vi "pmu_Build Time Quality (Std 2011).vi"(0 "reported GPS information":T1, 1 "max time error [s]":dbl=1e-07 format="%#_15f", 9 "system info in":refnum<class "PMU System Info.lvclass">, 11 "error in (no error)":errorcluster) -> (4 "reporting timing information":T2 {"PMU time quality" format="%.0b"; "time quality flag" format="%.0b"}, 10 "system info out":refnum<class "PMU System Info.lvclass">, 15 "error out":errorcluster)   [LabVIEW 2015, in "NI_EP_PMU.lvlib"]
doc: "Outputs time quality flag bits, according to IEEE Std C37.118."
uses:
  <vilib>/addons/Electrical Power/PMU/NI_EP_PMU.lvlib
  <vilib>/addons/Electrical Power/PMU/Common/Controls/pmu_Reporting Time Information (Std 2011).ctl
  <vilib>/addons/Electrical Power/PMU/Common/Classes/PMU System Info/PMU System Info.lvclass
  <vilib>/addons/Electrical Power/PMU/Common/Controls/pmu_GPS Info.ctl
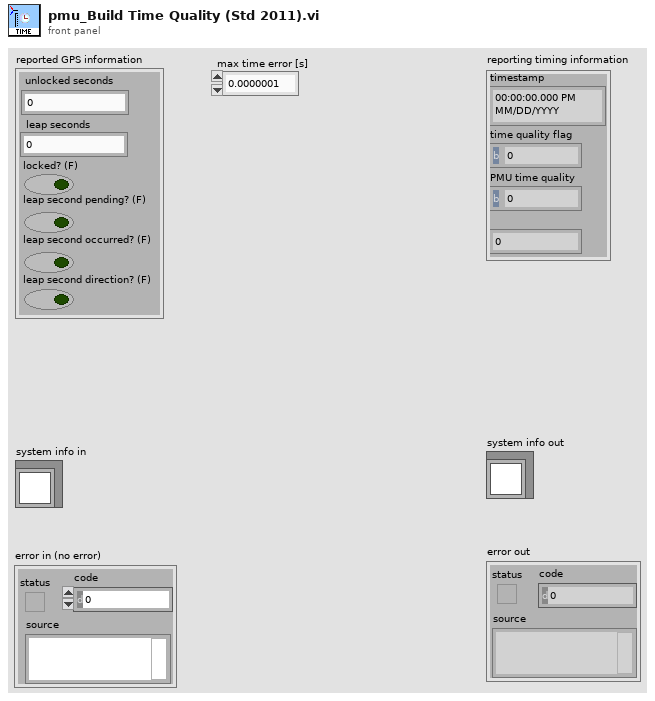
[diagram p1: front panel]
types:
  T1 = typedef "NI_EP_PMU.lvlib/pmu_GPS Info.ctl" = cluster{"unlocked seconds":u32, "leap seconds":i8, "locked? (F)":bool, "leap second pending? (F)":bool, "leap second occurred? (F)":bool, "leap second direction? (F)":bool}
  T2 = typedef "NI_EP_PMU.lvlib/pmu_Reporting Time Information (Std 2011).ctl" = cluster{"timestamp":timestamp, "time quality flag":u8, "PMU time quality":u8, "unlocked seconds":u32}
  T3 = cluster{"leap second pending":bool, "leap second direction":bool, "leap second occurred":bool}
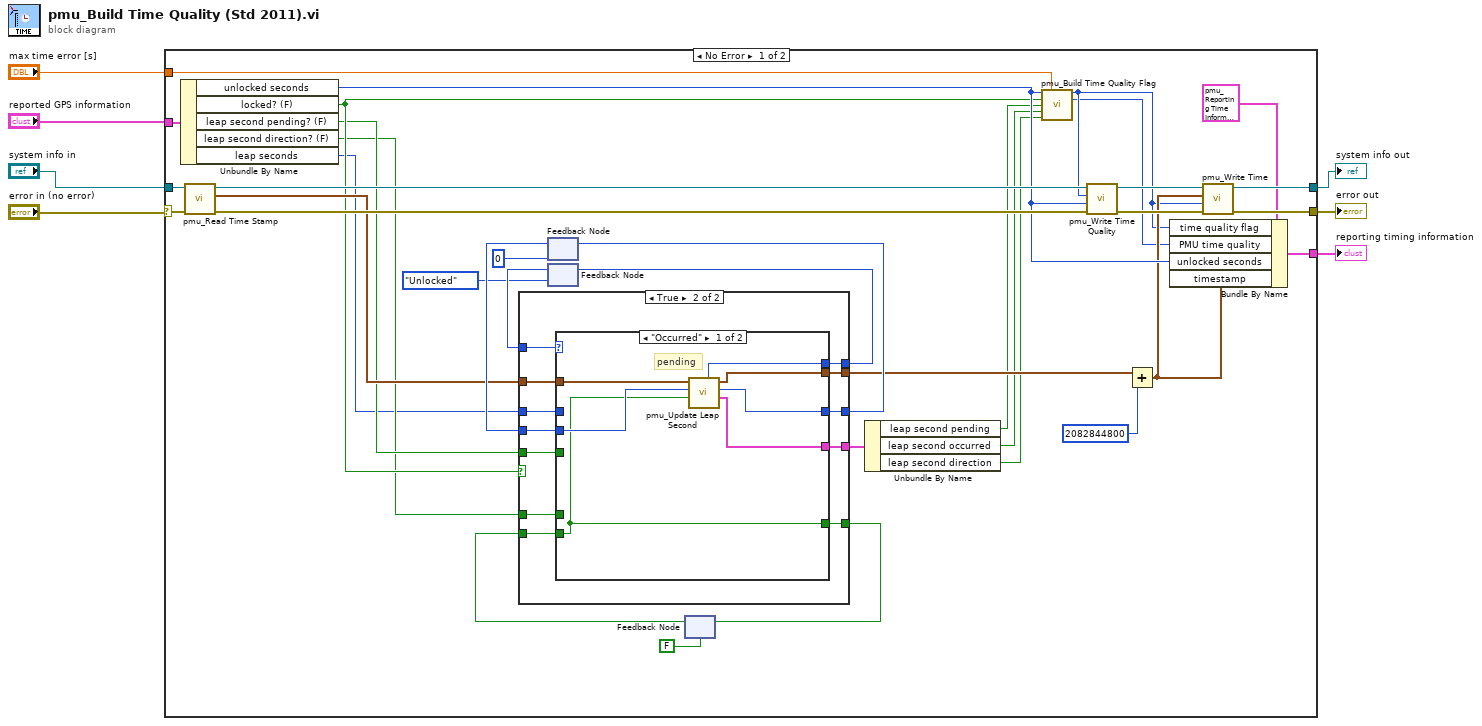
[diagram p0: block diagram]
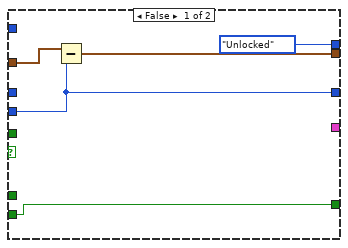
[diagram p2: hidden frame]
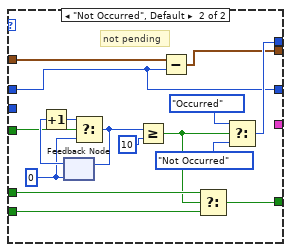
[diagram p3: hidden frame]
diagram:
  n1 = case shown="No Error" "error in (no error)" {
    selector: "error in (no error)" -> [w35 w84]
    tunnel: "system info in" -> [w36 _]
    tunnel: "max time error [s]" -> [w43 _]
    tunnel: [w41 w84] -> w6
    tunnel: [w40 _] -> w5
    tunnel: "reported GPS information" -> [w34 _]
    tunnel: [w31 _] -> w1
    frame No Error {
      n2 = Unbundle By Name(w34) -> ("unlocked seconds"=w32:u32, "locked? (F)"=w19:bool, "leap second pending? (F)"=w18:bool, "leap second direction? (F)"=w9:bool, "leap seconds"=w8:i8)
      n3 = call <vilib>:"pmu_Read Time Stamp.vi"("error in (no error)"=w35, "system info in"=w36) -> ("error out"=w37:errorcluster, "time stamp"=w25:timestamp, "system info out"=w38:refnum<class "PMU System Info.lvclass">)  [unwired: 7 in]
      n4 = feedback #1(i8 0 ("leap seconds")) -> (w29:i8)
      n5 = feedback #2(enum16{"Unlocked", "Not Occurred", "Occurred"}."Unlocked" ("f")) -> (w27:enum16{"Unlocked", "Not Occurred", "Occurred"})
      n6 = feedback #3(FALSE ("UTC offset valid? (F)")) -> (w16:bool)
      n7 = case shown="True" w19 {
        tunnel: w25 -> [w48 w60]
        tunnel: w8 -> [_ w49]
        tunnel: [w46 w59] -> w14
        tunnel: [w47 w56] -> w30
        tunnel: w29 -> [w47 w55]
        tunnel: w27 -> [_ w57]
        tunnel: [enum16{"Unlocked", "Not Occurred", "Occurred"}."Unlocked" w58] -> w26
        tunnel: w18 -> [_ w54]
        tunnel: w16 -> [w44 w53]
        tunnel: w9 -> [_ w52]
        tunnel: [w44 w51] -> w15
        tunnel: [_ w50] -> w13
        frame False {
          n8 = Subtract(x=w48, y=w47) -> (x-y=w46:timestamp)
        }
        frame True {
          n9 = case shown="\"Occurred\"" w57 {
            tunnel: w54 -> [_ w73]
            tunnel: w60 -> [w67 w83]
            tunnel: w55 -> [w66 _]
            tunnel: [w63 w76] -> w59
            tunnel: [w64 w80] -> w58
            tunnel: [w62 w75] -> w56
            tunnel: w53 -> [w65 w78]
            tunnel: w52 -> [_ w79]
            tunnel: [w65 w77] -> w51
            tunnel: [w61 _] -> w50
            tunnel: w49 -> [_ w75]
            frame "Occurred" {
              # "pending"
              n10 = call <vilib>:"pmu_Update Leap Second.vi"("leap second direction"=w65, "leap seconds"=w66, "time stamp"=w67) -> ("leap second status"=w61:T3, "leap seconds out"=w62:i8, "time stamp out"=w63:timestamp, "status"=w64:enum16{"Unlocked", "Not Occurred", "Occurred"})  [unwired: 5 in]
            }
            frame "Not Occurred", Default {
              w71 = u8 0 ("leap seconds")
              # "not pending"
              n11 = feedback #4(w71) -> (w74:u8)
              n12 = Increment(x=w74) -> (x+1=w72:u8)
              n13 = Select(t=w72, s=w73, f=w71) -> (s? t:f=w70:u8)
              n14 = feedback-in #4(w70) -> ()
              n15 = Greater Or Equal?(x=w70, y=u8 10 ("leap seconds")) -> (x >= y?=w68:bool)
              n16 = Subtract(x=w83, y=w75) -> (x-y=w76:timestamp)
              n17 = Select(t=w79, s=w68, f=w78) -> (s? t:f=w77:bool)
              n18 = Select(t=enum16{"Unlocked", "Not Occurred", "Occurred"}."Occurred" ("f"), s=w68, f=enum16{"Unlocked", "Not Occurred", "Occurred"}."Not Occurred") -> (s? t:f=w80:enum16{"Unlocked", "Not Occurred", "Occurred"})
            }
          }
        }
      }
      n19 = feedback-in #1(w30) -> ()
      n20 = feedback-in #2(w26) -> ()
      n21 = feedback-in #3(w15) -> ()
      n22 = Unbundle By Name(w13) -> ("leap second pending"=w12:bool, "leap second occurred"=w11:bool, "leap second direction"=w10:bool)
      n23 = call <vilib>:"pmu_Build Time Quality Flag.vi"("unlocked seconds"=w32, "synchronization error (s)"=w43, "locked?"=w19, "leap second pending"=w12, "leap second occurred"=w11, "leap second direction"=w10) -> ("time quality flag"=w21:u8, "PMU time quality"=w20:u8)  [unwired: 8 in]
      n24 = call <vilib>:"pmu_Write Time Quality.vi"("error in (no error)"=w37, "unlocked time"=w32, "time quality flag"=w21, "system info in"=w38) -> ("error out"=w42:errorcluster, "system info out"=w39:refnum<class "PMU System Info.lvclass">)  [unwired: 6 in]
      n25 = Add(x=w14, y=u32 2082844800 ("unsigned 32bit integer")) -> (x+y=w23:timestamp)
      n26 = Bundle By Name(cluster=T2 {"timestamp"=timestamp(0 s since 1904-01-01), "time quality flag"=0, "PMU time quality"=0, "unlocked seconds"=0} ("reporting timing information"), "time quality flag"=w21, "PMU time quality"=w20, "unlocked seconds"=w32, "timestamp"=w23) -> (w31:T2)
      n27 = call <vilib>:"pmu_Write Time .vi"("error in (no error)"=w42, "time quality"=w21, "time stamp"=w23, "system info in"=w39) -> ("error out"=w41:errorcluster, "system info out"=w40:refnum<class "PMU System Info.lvclass">)  [unwired: 6 in]
    }
    frame Error {
    }
  }
  "reporting timing information" <- w1
  "error out" <- w6
  "system info out" <- w5
